vi "S2DS_Set Scan type string (SubVI).vi"(11 "All channel parameters (in)":T1 {"Scan parameters"."Y data taking" items=["in both direction", "in up direction only", "in down direction only"]; "Scan parameters"."X data taking" items=["in both direction", "in up direction only", "in down direction only"]}) -> (0 "Scan type string":string[](array[string]), 3 "X Y Channel names (out)":string[](array[string]))   [LabVIEW 2025]
uses:
  TYPE DEFS/S2DS_All Channel Parameters.ctl
  TYPE DEFS/S2DS_WC info.ctl
  TYPE DEFS/S2DS_Single WC info.ctl
  TYPE DEFS/S2DS_RC info.ctl
  TYPE DEFS/S2DS_Single RC info.ctl
  TYPE DEFS/S2DS_DAC info new.ctl
  TYPE DEFS/S2DS_Single DC info.ctl
  TYPE DEFS/S2DS_Array Inst Info.ctl
  TYPE DEFS/S2DS_Sweep Info.ctl
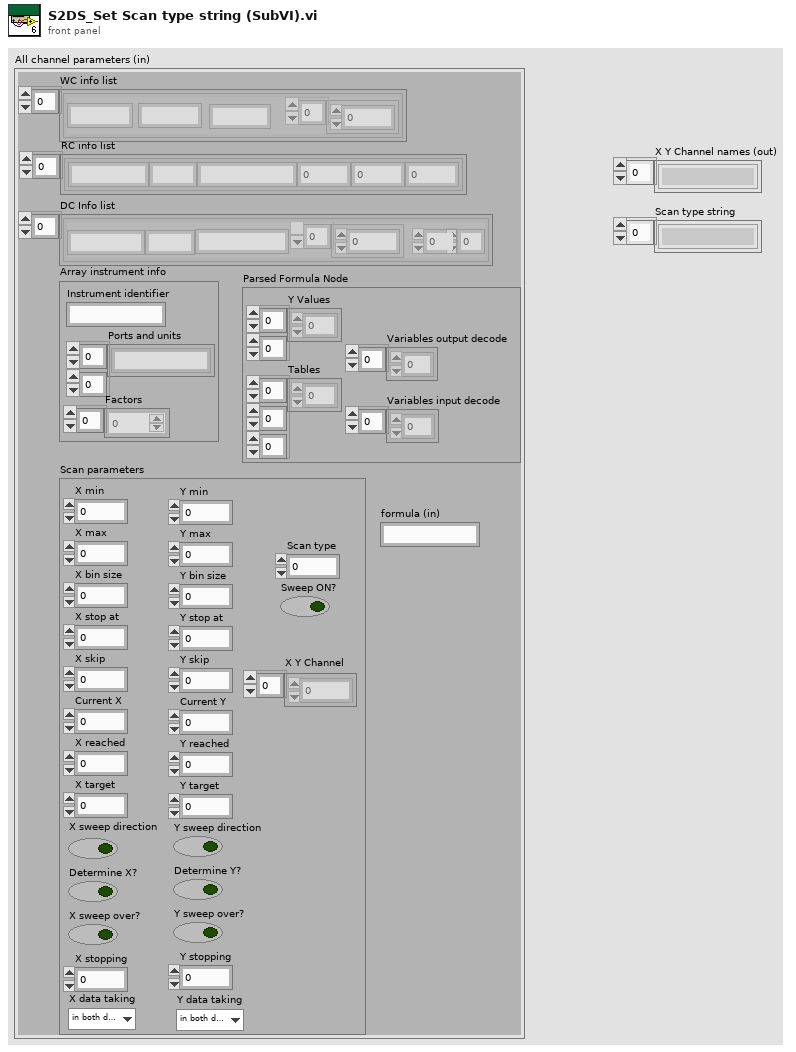
[diagram p1: front panel]
types:
  T1 = typedef "S2DS_All Channel Parameters.ctl" = cluster{"WC info list":T2, "RC info list":T4, "DC Info list":T6, "Array instrument info":T8, "Scan parameters":T9, "Parsed Formula Node":cluster{"Y Values":dbl[][], "Tables":i32[][][], "Variables input decode":i32[], "Variables output decode":i32[]}, "formula (in)":string}
  T2 = typedef "S2DS_WC info.ctl" = T3[]
  T3 = typedef "S2DS_Single WC info.ctl" = cluster{"Instrument identifier":string, "Write channel parameters":dbl[], "Name":string, "Unit":string}
  T4 = typedef "S2DS_RC info.ctl" = T5[]
  T5 = typedef "S2DS_Single RC info.ctl" = cluster{"Instrument identifier":string, "Factor":dbl, "Averaging":i32, "Wait (ms)":i32, "Unit":string, "Name":string}
  T6 = typedef "S2DS_DAC info new.ctl" = T7[]
  T7 = typedef "S2DS_Single DC info.ctl" = cluster{"Operation identifier":string, "DC parameters":dbl[], "U":i32, "V":i32, "Name":string, "Unit":string}
  T8 = typedef "S2DS_Array Inst Info.ctl" = cluster{"Instrument identifier":string, "Ports and units":string[][], "Factors":dbl[]}
  T9 = typedef "S2DS_Sweep Info.ctl" = cluster{"X min":ext, "X max":dbl, "Y min":dbl, "Y max":dbl, "X bin size":dbl, "Y bin size":dbl, "X stop at":dbl, "Y stop at":dbl, "X skip":u64, "Y skip":u64, "Current X":dbl, "Current Y":dbl, "X reached":i32, "Y reached":i32, "X target":dbl, "Y target":dbl, "Sweep ON?":bool, "X sweep direction":bool, "Y sweep direction":bool, "Determine X?":bool, "Determine Y?":bool, "X sweep over?":bool, "Y sweep over?":bool, "Scan type":i32, "X stopping":i32, "Y stopping":i32, "X Y Channel":u16[], "X data taking":u16, "Y data taking":u16}
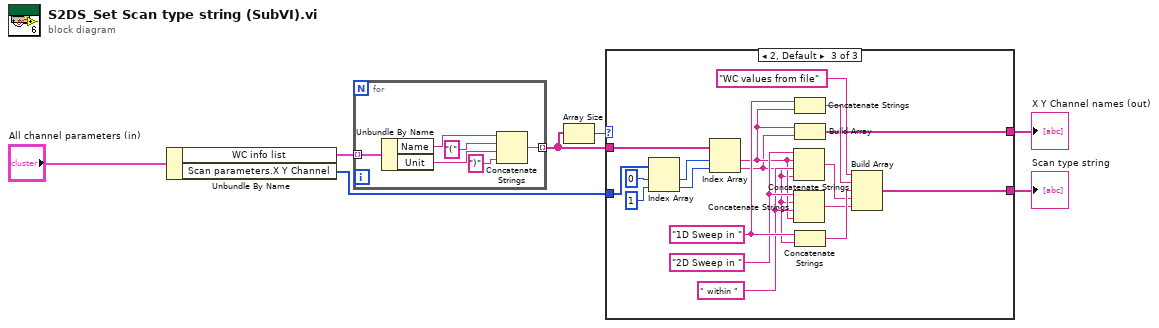
[diagram p0: block diagram]
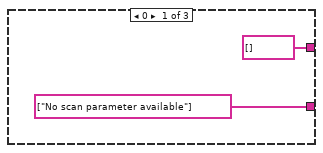
[diagram p2: hidden frame]
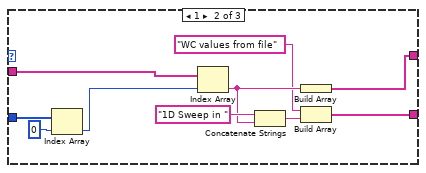
[diagram p3: hidden frame]
diagram:
  n1 = Unbundle By Name("All channel parameters (in)") -> ("WC info list"=w5:T2, "Scan parameters.X Y Channel"=w1:u16[])
  n2 = for {
    tunnel: w5 -> [w13] mode=indexing
    tunnel: [w8] -> w4 mode=indexing
    n3 = Unbundle By Name(w13) -> ("Name"=w12:string, "Unit"=w10:string)
    n4 = Concatenate Strings(w12, "(" ("string"), w10, ")" ("string")) -> (w8:string)
  }
  n5 = Array Size(array=w4) -> (size(s)=w3:i32)
  n6 = case shown="2, Default" w3 {
    tunnel: w4 -> [_ w25 w43]
    tunnel: [string[] ["No scan parameter available"] w22 w35] -> w7
    tunnel: w1 -> [_ w19 w31]
    tunnel: [string[] [] w20 w32] -> w2
    frame 0 {
    }
    frame 1 {
      n7 = Index Array(array=w19, index=0) -> (element=w18:u16)
      n8 = Index Array(array=w25, index=w18) -> (element=w21:string)
      n9 = Concatenate Strings("1D Sweep in ", w21) -> (w23:string)
      n10 = Build Array(w21) -> (w20:string[])
      n11 = Build Array("WC values from file" ("element"), w23) -> (w22:string[])
    }
    frame 2, Default {
      w40 = " within "
      w41 = "2D Sweep in "
      w42 = "1D Sweep in "
      n12 = Index Array(array=w31, index #1=0 ("index"), index #2=1 ("index")) -> (element #1=w28:u16, element #2=w27:u16)
      n13 = Index Array(array=w43, index #1=w28, index #2=w27) -> (element #1=w34:string, element #2=w33:string)
      n14 = Concatenate Strings(w41, w34, w40, w33) -> (w37:string)
      n15 = Concatenate Strings(w41, w33, w40, w34) -> (w36:string)
      n16 = Concatenate Strings(w42, w34) -> (w39:string)
      n17 = Build Array(w34, w33) -> (w32:string[])
      n18 = Concatenate Strings(w42, w33) -> (w38:string)
      n19 = Build Array("WC values from file" ("element"), w39, w38, w37, w36) -> (w35:string[])
    }
  }
  "Scan type string" <- w7
  "X Y Channel names (out)" <- w2
